vi "binary to decimal or decimal to bnary.vi"() -> ()   [LabVIEW 2013]
panel:
  out "Boolean 8":bool
  out "Boolean 7":bool
  out "Boolean 6":bool
  out "Boolean 5":bool
  in  "Numeric 9":dbl
  in  "Numeric 8":dbl
  in  "Numeric 7":dbl
  in  "Numeric 6":dbl
  out "Numeric 5":dbl
  out "Numeric 4":dbl
  out "Numeric 3":dbl
  out "Numeric 2":dbl
  out "Numeric":dbl
  in  "Boolean 4":bool
  in  "Boolean 3":bool
  in  "Boolean 2":bool
  in  "Boolean":bool
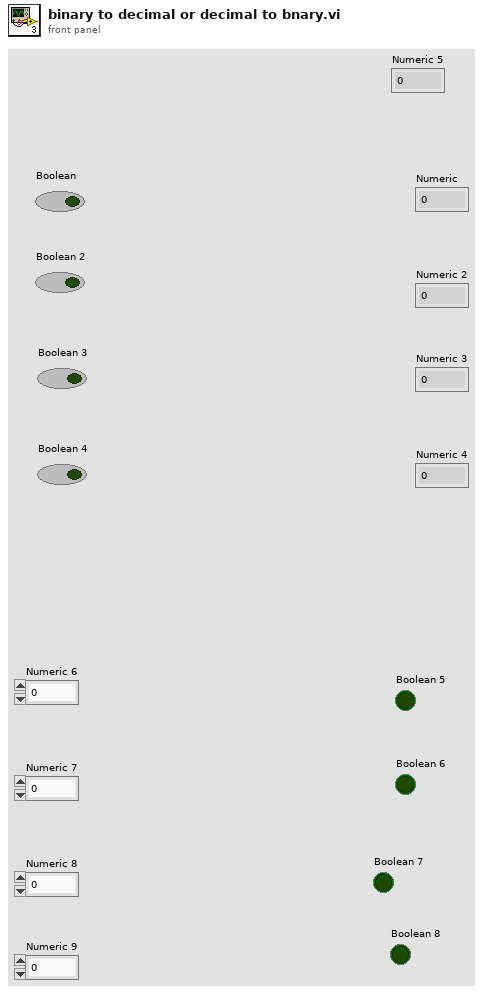
[diagram p1: front panel]
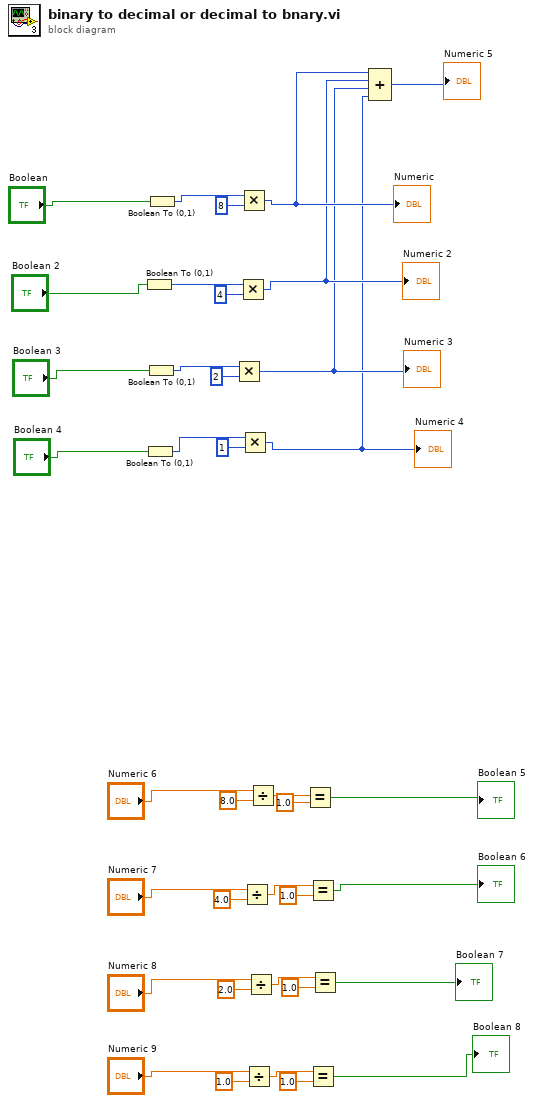
[diagram p0: block diagram]
diagram:
  n1 = Boolean To (0,1)(Boolean="Boolean 2") -> (0, 1=w36:i16)
  n2 = Boolean To (0,1)(Boolean="Boolean 4") -> (0, 1=w34:i16)
  n3 = Boolean To (0,1)(Boolean="Boolean 3") -> (0, 1=w35:i16)
  n4 = Boolean To (0,1)(Boolean="Boolean") -> (0, 1=w37:i16)
  n5 = Multiply(x=w35, y=i16 2) -> (x*y=w23:i16)
  "Numeric 3" <- w23
  n6 = Multiply(x=w36, y=i16 4) -> (x*y=w24:i16)
  "Numeric 2" <- w24
  n7 = Multiply(x=w37, y=i16 8) -> (x*y=w25:i16)
  "Numeric" <- w25
  n8 = Multiply(x=w34, y=i16 1) -> (x*y=w22:i16)
  "Numeric 4" <- w22
  n9 = Divide(x="Numeric 7", y=4.0) -> (x/y=w9:dbl)
  n10 = Divide(x="Numeric 9", y=1.0) -> (x/y=w7:dbl)
  n11 = Divide(x="Numeric 8", y=2.0) -> (x/y=w8:dbl)
  n12 = Divide(x="Numeric 6", y=8.0) -> (x/y=w18:dbl)
  n13 = Equal?(x=w18, y=1.0) -> (x = y?=→"Boolean 5":bool)
  n14 = Equal?(x=w9, y=1.0) -> (x = y?=→"Boolean 6":bool)
  n15 = Equal?(x=w7, y=1.0) -> (x = y?=→"Boolean 8":bool)
  n16 = Equal?(x=w8, y=1.0) -> (x = y?=→"Boolean 7":bool)
  n17 = Compound Arithmetic op=ADD(w25, w24, w23, w22) -> (→"Numeric 5":i16)
